vi "Scan Setup.vi"(8 "error in (no error)":errorcluster, 11 "Reader in":refnum<class "Reader.lvclass">) -> (0 "error out":errorcluster, 3 "Reader out":refnum<class "Reader.lvclass">)   [LabVIEW 2009, in "Reader.lvclass"]
doc: "(Dynamic) Send commands to configure the instrument based on the class member fields."
uses:
  Reader.lvclass
  Reader.lvclass/Reader.ctl
  Instruments/Utility Classes/Readable/Readable.lvclass
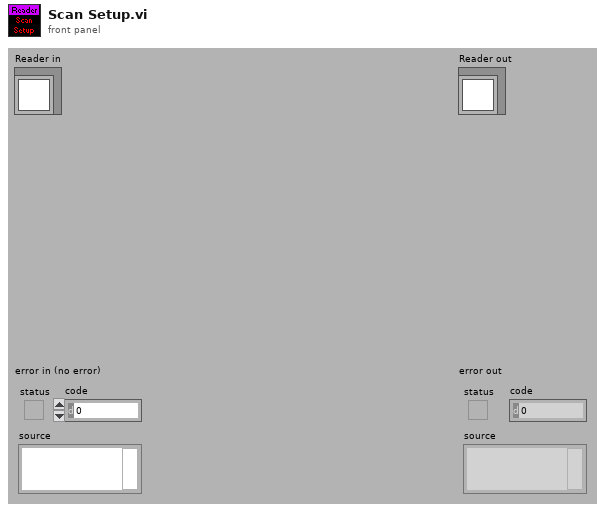
[diagram p1: front panel]
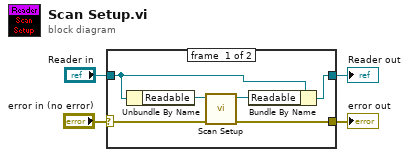
[diagram p0: block diagram]
diagram:
  n1 = case shown="No Error" "error in (no error)" {
    selector: "error in (no error)" -> [w6 w12]
    tunnel: [w5 w12] -> w3
    tunnel: [w9 w11] -> w1
    tunnel: "Reader in" -> [w10 w11]
    frame #0 {
      n2 = Unbundle By Name(w10) -> ("Readable"=w8:refnum<class "Readable.lvclass">)
      n3 = call-dynamic "Scan Setup.vi"("error in (no error)"=w6, "Instrument in"=w8) -> ("error out"=w5:errorcluster, "Instrument out"=w7:refnum<class "Readable.lvclass">)  [unwired: 8 out]
      n4 = Bundle By Name(cluster=w10, "Readable"=w7) -> (w9:refnum<class "Reader.lvclass">)
    }
    frame #1 {
    }
  }
  "error out" <- w3
  "Reader out" <- w1
